vi "test_TxUDPBlockWrite.vi"() -> ()   [LabVIEW 2020]
uses:
  <instrlib>/AIM GmbH/_AIM 664/_controls/port_configuration.ctl
  <instrlib>/AIM GmbH/_AIM 664/_controls/port_speed.ctl
  <instrlib>/AIM GmbH/_AIM 664/_controls/comm_config_vl_tx.ctl
  <instrlib>/AIM GmbH/_AIM 664/_controls/comm_udp_tx.ctl
  <instrlib>/AIM GmbH/_AIM 664/helpers/EthFrameManagement/controls/arinc664_mac_src_info.ctl
  <instrlib>/AIM GmbH/_AIM 664/_controls/comm_computedMAC-IP.ctl
  <instrlib>/AIM GmbH/_AIM 664/bsp/Fdx Create Session (Tx-UDP Port-Oriented).vi
  <instrlib>/AIM GmbH/_AIM 664/bsp/Transmit/FdxCreateTxVL.vi
  <instrlib>/AIM GmbH/_AIM 664/bsp/Fdx Create UDP Port (TX-CommPort).vi
  <instrlib>/AIM GmbH/_AIM 664/bsp/Fdx Start (Tx).vi
  <instrlib>/AIM GmbH/_AIM 664/bsp/Fdx Stop (Tx).vi
  <instrlib>/AIM GmbH/_AIM 664/AIM664LV.lvlib
  BlockMessage/UdpBlockMessage.lvlib
  <instrlib>/AIM GmbH/_AIM 664/bsp/Fdx Create Session (Generic-Board).vi
  <instrlib>/AIM GmbH/_AIM 664/helpers/EthFrameManagement/EthFrameManagement.lvlib
panel:
  out "MsgCountOut":u32
  out "MsgCount 2":u32=2
  out "UdpBlockWriteResultArray":u32[](array[numeric])
  out "Waveform Chart":u32(graph)
  out "CurrentIndex":u32
  out "IndexCycleCount":u32
  out "MsgCount":u32
  out "TxStatus":T1 {"TransmitMode" items=["FDX_TX_GENERIC", "FDX_TX_REPLAY", "FDX_TX_INDIVIDUAL"]; "TxStatus" items=["FDX_STAT_STOP", "FDX_STAT_RUN", "FDX_STAT_ERROR", "FDX_STAT_WAIT_F_TRIG"]}
  in  "stop":bool
  out "Array":T2[](array[typedef]) {"MACsrc" format="%.0x"}
  out "Buf":u8[](array[numeric]) format="%.0x"
  in  "Buf Lenght":i32=512
  in  "VlTx":T3={"domainID"=1, "sideID"=1, "locationID"=1, "interfaceID"=1}
  in  "CommPort Config":T4[](array[typedef])=[{"PortType"=enum."FDX_UDP_SAMPLING", "partitionID"=1, "SubVlId"=1, "UdpSrcPort"=24, "UdpDstPort"=23, "SampleRateMs"=64.0, "UdpNumBufMessages"=1, "UdpMaxMessageSize"=512}, {"PortType"=enum."FDX_UDP_SAMPLING", "partitionID"=2, "SubVlId"=2, "UdpSrcPort"=34, "UdpDstPort"=33, "SampleRateMs"=64.0, "UdpNumBufMessages"=1, "UdpMaxMessageSize"=512}, {"PortType"=enum."FDX_UDP_SAMPLING", "partitionID"=3, "SubVlId"=3, "UdpSrcPort"=44, "UdpDstPort"=43, "SampleRateMs"=64.0, "UdpNumBufMessages"=1, "UdpMaxMessageSize"=512}, {"PortType"=enum."FDX_UDP_SAMPLING", "partitionID"=3, "SubVlId"=4, "UdpSrcPort"=54, "UdpDstPort"=53, "SampleRateMs"=64.0, "UdpNumBufMessages"=1, "UdpMaxMessageSize"=512}]
  in  "VL Config":T5[](array[typedef])=[{"VlId"=60, "NumOfSubVl"=4, "rate ms [Bag]"=64, "domainID"=1, "sideID"=1, "locationID"=1, "interfaceID"=1, "NetSelect"=3, "Skew"=0, "MaxFrameLength"=1518, "FrameBufferSize"=0}] {"NetSelect" items=["FDX_TX_FRAME_DLY_A"=0, "FDX_TX_FRAME_DLY_B"=1, "FDX_TX_FRAME_BOTH "=3, "FDX_TX_FRAME_ONLY_A"=4, "FDX_TX_FRAME_ONLY_B "=5]; "interfaceID" format="%.0b"}
  in  "PortMap":u32=1
  out "PortInitOut":T6 {"PortConfig" items=["FDX_SINGLE", "FDX_REDUNDANT"]}
  in  "port":u32
  in  "PortSpeed":T7[](array[typedef])=[0, 0] items=["FDX_100MBIT"=0, "FDX_10MBIT"=1, "FDX_1000MBIT"=5, "FDX_AUTO_100MBIT"=2, "FDX_AUTO_10MBIT"=3]
  in  "PortConfig":T8[](array[typedef])=[0, 0] items=["FDX_SINGLE", "FDX_REDUNDANT"]
  out "timed out":bool
  out "good link":bool
  out "error out":errorcluster
  in  "board":u32
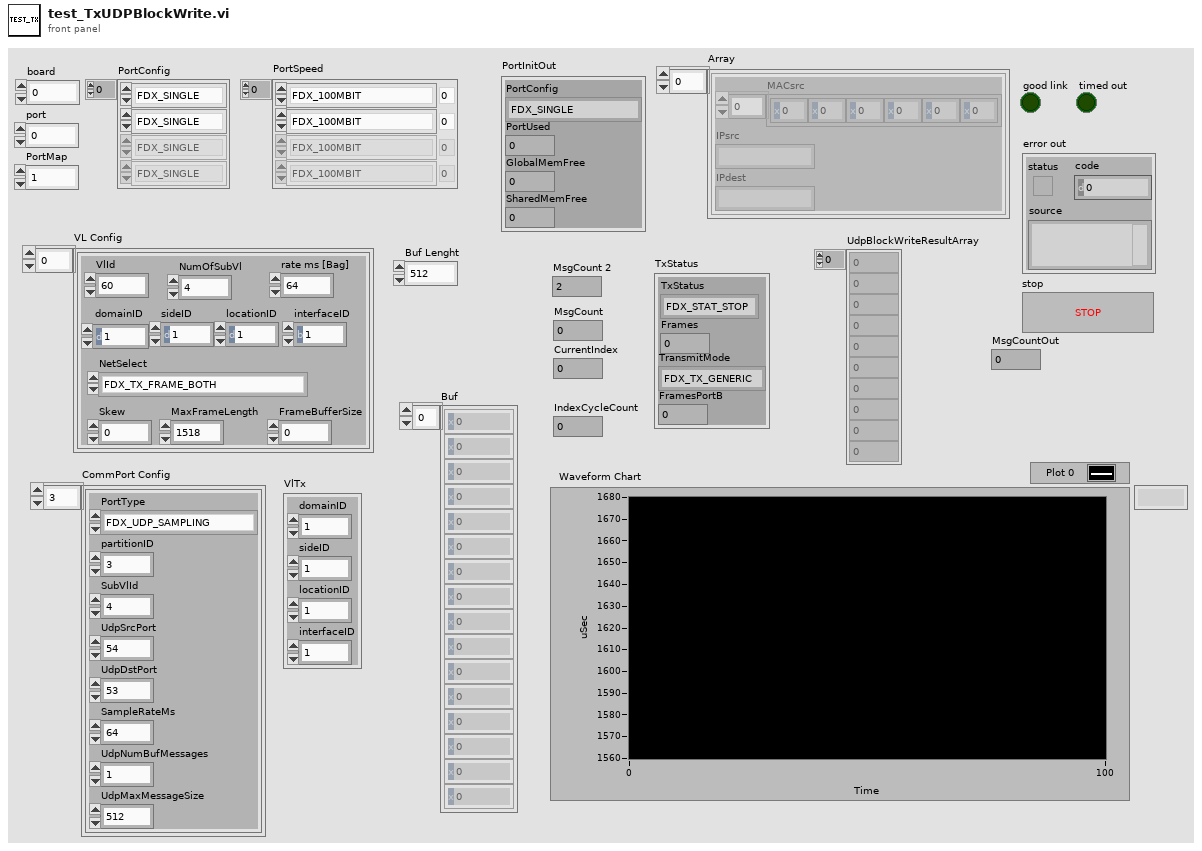
[diagram p1: front panel]
types:
  T1 = cluster{"TxStatus":u32, "Frames":u32, "TransmitMode":u32, "FramesPortB":u32}
  T2 = typedef "AIM664LV.lvlib/comm_computedMAC-IP.ctl" = cluster{"MACsrc":u8[], "IPsrc":string, "IPdest":string}
  T3 = typedef "EthFrameManagement.lvlib/arinc664_mac_src_info.ctl" = cluster{"domainID":u8, "sideID":u8, "locationID":u8, "interfaceID":u8}
  T4 = typedef "AIM664LV.lvlib/comm_udp_tx.ctl" = cluster{"PortType":enum16{"FDX_UDP_SAMPLING", "FDX_UDP_QUEUING"}, "partitionID":u8, "SubVlId":u8, "UdpSrcPort":u16, "UdpDstPort":u16, "SampleRateMs":dbl, "UdpNumBufMessages":u32, "UdpMaxMessageSize":u32}
  T5 = typedef "AIM664LV.lvlib/comm_config_vl_tx.ctl" = cluster{"VlId":u16, "NumOfSubVl":u16, "rate ms [Bag]":u32, "domainID":u8, "sideID":u8, "locationID":u8, "interfaceID":u8, "NetSelect":u32, "Skew":u32, "MaxFrameLength":u32, "FrameBufferSize":u32}
  T6 = cluster{"PortConfig":u32, "PortUsed":u32, "GlobalMemFree":u32, "SharedMemFree":u32}
  T7 = typedef "AIM664LV.lvlib/port_speed.ctl" = u32
  T8 = typedef "AIM664LV.lvlib/port_configuration.ctl" = u32
  T9 = typedef "UdpBlockMessage.lvlib/ubm_value_type.ctl" = cluster{"ul_ByteCount":u32, "ul_UdpHandle":u32, "write index":u32}
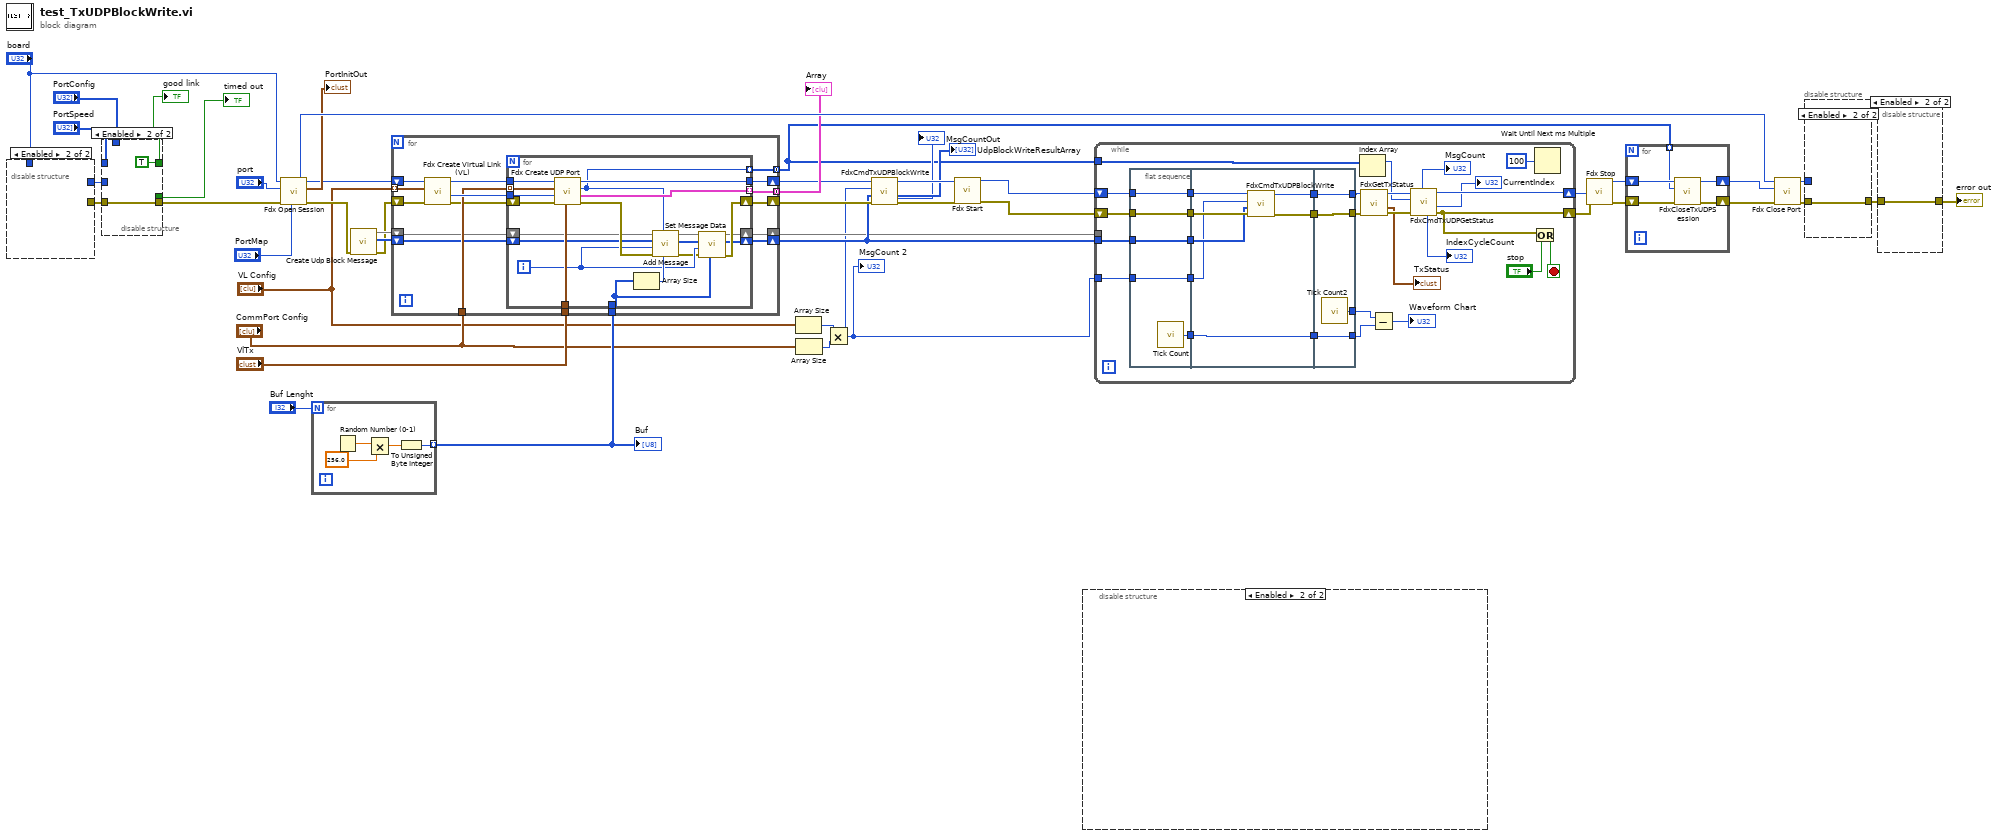
[diagram p0: block diagram]
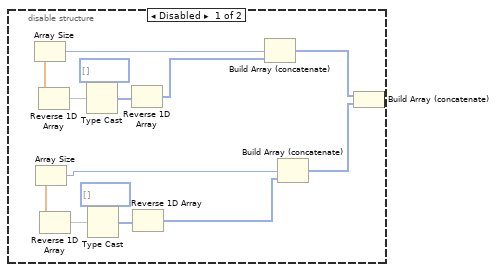
[diagram p2: hidden frame]
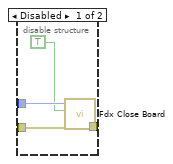
[diagram p3: hidden frame]
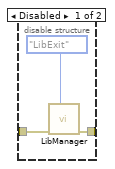
[diagram p4: hidden frame]
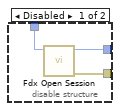
[diagram p5: hidden frame]
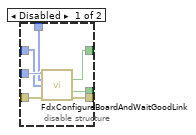
[diagram p6: hidden frame]
diagram:
  n1 = disable-structure shown="Enabled" {
    disable-tunnel: [w50 _] -> w47
    disable-tunnel: [w49 _] -> w46
    disable-tunnel: "board" -> [w48 _]
    frame Disabled {
      n2 = call-poly <instrlib>:"Fdx Open Session.vi"("board"=w48) -> ("error out"=w49:errorcluster, "InstrumentHandle_board out"=w50:u32)  [unwired: 8 in, 1 out]
    }
    frame Enabled {
    }
  }
  n3 = disable-structure shown="Enabled" {
    disable-tunnel: w47 -> [w57 _]
    disable-tunnel: w46 -> [w56 w59]
    disable-tunnel: [w55 TRUE ("good link")] -> w45
    disable-tunnel: [w54 _] -> w44
    disable-tunnel: "PortConfig" -> [w53 _]
    disable-tunnel: "PortSpeed" -> [w52 _]
    disable-tunnel: [w51 w59] -> w41
    frame Disabled {
      n4 = call <instrlib>:"FdxConfigureBoardAndWaitGoodLink.vi"("InstrumentHandle_board in"=w57, "PortConfig"=w53, "PortSpeed"=w52, "error in"=w56) -> ("good link"=w55:bool, "timed out"=w54:bool, "error out"=w51:errorcluster)  [unwired: 8 in, 1 out]
    }
    frame Enabled {
    }
  }
  "good link" <- w45
  "timed out" <- w44
  n5 = call-poly <instrlib>:"Fdx Open Session.vi"("PortMap"="PortMap", "error in (no error)"=w41, "port"="port", "board"="board") -> ("error out"=w7:errorcluster, "PortInitOut"=→"PortInitOut":T6, "port handle out"=w31:u32, "InstrumentHandle_board out"=w36:u32)  [unwired: 3 in, 1 out]
  n6 = for {
    N: "Buf Lenght" -> [_]
    tunnel: [w60] -> w12 mode=indexing
    n7 = Random Number (0-1)() -> (number: 0 to 1=w63:dbl)
    n8 = Multiply(x=w63, y=256.0) -> (x*y=w61:dbl)
    n9 = To Unsigned Byte Integer(number=w61) -> (unsigned 8bit integer=w60:u8)
  }
  "Buf" <- w12
  n10 = call "Create Udp Block Message.vi"("error in (no error)"=w7) -> ("error out"=w4:errorcluster, "Message Block Array"=w5:u32[], "Udp Block Message Map"=w6:map{i32, T9})  [unwired: 8 in]
  n11 = for {
    tunnel: "VL Config" -> [w78] mode=indexing
    tunnel: "VlTx" -> [w75]
    tunnel: [w74] -> w29 mode=concatenating
    tunnel: [w71] -> w13 mode=concatenating
    tunnel: w12 -> [w70]
    tunnel: "CommPort Config" -> [w67]
    shift-right: [w72] -> w18
    shift-left: w4 -> [w80]
    shift-right: [w73] -> w20
    shift-left: w31 -> [w79]
    shift-right: [w68] -> w10
    shift-left: w6 -> [w65]
    shift-right: [w69] -> w11
    shift-left: w5 -> [w64]
    n12 = call-poly <instrlib>:"Fdx Create Virtual Link (VL).vi"("error in (no error)"=w80, "VL Config"=w78, "InstrumentHandle in"=w79) -> ("error out"=w66:errorcluster, "VlId"=w76:u16, "InstrumentHandle out"=w77:u32)  [unwired: 6 in]
    n13 = for {
      tunnel: w77 -> [w100]
      tunnel: w76 -> [w99]
      tunnel: w67 -> [w97] mode=indexing
      tunnel: w75 -> [w96]
      tunnel: [w95] -> w74 mode=indexing
      tunnel: [w94] -> w73
      tunnel: [w90] -> w71 mode=indexing
      shift-right: [w83] -> w72
      shift-left: w66 -> [w98]
      shift-right: [w81] -> w69
      shift-left: w64 -> [w89]
      shift-right: [w82] -> w68
      shift-left: w65 -> [w92]
      tunnel: w70 -> [w88]
      i -> [w87]
      n14 = call-poly <instrlib>:"Fdx Create UDP Port.vi"("VlTx"=w96, "error in"=w98, "VlId"=w99, "CommPort Config"=w97, "port handle in"=w100) -> ("error out"=w93:errorcluster, "computedAddresses"=w95:T2, "commPort handle out"=w90:u32, "port handle out"=w94:u32)  [unwired: 3 in]
      n15 = Array Size(array=w88) -> (size(s)=w91:i32)
      n16 = call "Add Message.vi"("ul_ByteCount"=w91, "ul_UdpHandle"=w90, "error in (no error)"=w93, "index"=w87, "Message Block Array in"=w89, "Udp Block Message Map in"=w92) -> ("error out"=w84:errorcluster, "Message Block Array out"=w85:u32[], "Udp Block Message Map out"=w86:map{i32, T9})  [unwired: 3 in]
      n17 = call "Set Message Data.vi"("Data in"=w88, "error in (no error)"=w84, "index"=w87, "Message Block Array in"=w85, "Udp Block Message Map in"=w86) -> ("error out"=w83:errorcluster, "Message Block Array out"=w81:u32[], "Udp Block Message Map out"=w82:map{i32, T9})  [unwired: 4 in]
    }
  }
  "Array" <- w29
  n18 = Array Size(array="VL Config") -> (size(s)=w1:i32)
  n19 = Array Size(array="CommPort Config") -> (size(s)=w9:i32)
  n20 = Multiply(x=w1, y=w9) -> (x*y=w2:i32)
  "MsgCount 2" <- w2
  n21 = call <instrlib>:"FdxCmdTxUDPBlockWrite.vi"("error in"=w18, "UdpBlockWriteMsgArray"=w11, "MsgCount"=w2, "InstrumentHandle"=w20) -> ("error out"=w17:errorcluster, "UdpBlockWriteResultArray"=→"UdpBlockWriteResultArray":u32[], "InstrumentHandle"=w19:u32, "MsgCountOut"=→"MsgCountOut":u32)  [unwired: 3 in, 1 out]
  n22 = call-poly <instrlib>:"Fdx Start.vi"("error in"=w17, "InstrumentHandle_port in"=w19) -> ("error out"=w28:errorcluster, "InstrumentHandle_port out"=w27:u32)  [unwired: 8 in]
  n23 = disable-structure shown="Enabled" {
    frame Disabled {
      n24 = Array Size() -> (array=w110:dbl[], size(s)=w115:i32)
      n25 = Reverse 1D Array() -> (array=w101:ext[], reversed array=w105:ext[])
      n26 = Array Size(array=w101) -> (size(s)=w102:i32)
      n27 = Reverse 1D Array(array=w110) -> (reversed array=w107:ext[])
      n28 = Type Cast(type=u32[] [] ("Buf"), x=w105) -> (*(type *) &x=w104:u32[])
      n29 = Type Cast(type=u32[] [] ("Buf"), x=w107) -> (*(type *) &x=w108:u32[])
      n30 = Reverse 1D Array(array=w104) -> (reversed array=w106:u32[])
      n31 = Reverse 1D Array(array=w108) -> (reversed array=w116:u32[])
      n32 = Build Array (concatenate)(w102, w106) -> (w111:u32[], w113:u32)
      n33 = Build Array (concatenate)(w115, w116) -> (w112:u32[], w114:u32)
      n34 = Build Array (concatenate)(w111, w112) -> ()  [unwired: 1 out]
    }
    frame Enabled {
    }
  }
  n35 = while {
    shift-right: [w140] -> w25
    shift-left: w27 -> [w134]
    shift-right: [w141] -> w26
    shift-left: w28 -> [w130]
    tunnel: w13 -> [w122]
    tunnel: w11 -> [w119]
    tunnel: w10 -> [_]
    tunnel: w2 -> [w117]
    stop <- w144 stop-if-true
    n36 = flat-sequence {
      tunnel: [w151] -> w135
      tunnel: w134 -> [w151]
      tunnel: [w150] -> w131
      tunnel: w130 -> [w150]
      tunnel: [w149] -> w128
      tunnel: [w148] -> w120
      tunnel: w119 -> [w148]
      tunnel: [w147] -> w118
      tunnel: w117 -> [w147]
      tunnel: w135 -> [w157]
      tunnel: [w154] -> w132
      tunnel: w131 -> [w156]
      tunnel: [w158] -> w129
      tunnel: w128 -> [w158]
      tunnel: [w155] -> w123
      tunnel: w120 -> [w153]
      tunnel: w118 -> [w152]
      tunnel: [w162] -> w133
      tunnel: w132 -> [w162]
      tunnel: [w161] -> w127
      tunnel: [w160] -> w126
      tunnel: w129 -> [w160]
      tunnel: [w159] -> w124
      tunnel: w123 -> [w159]
      frame #0 {
        n37 = call "Tick Count"() -> ("Tick Count(uSec)"=w149:u32)
      }
      frame #1 {
        n38 = call <instrlib>:"FdxCmdTxUDPBlockWrite.vi"("error in"=w156, "UdpBlockWriteMsgArray"=w153, "MsgCount"=w152, "InstrumentHandle"=w157) -> ("error out"=w155:errorcluster, "InstrumentHandle"=w154:u32)  [unwired: 3 in, 3 out]
      }
      frame #2 {
        n39 = call "Tick Count2"() -> ("Tick Count(uSec)"=w161:u32)
      }
    }
    n40 = Index Array(array=w122) -> (element=w121:u32)  [unwired: 1 in]
    n41 = call <instrlib>:"FdxGetTxStatus.vi"("error in"=w124, "InstrumentHandle_port"=w133) -> ("error out"=w143:errorcluster, "TxStatus"=→"TxStatus":T1, "InstrumentHandle_port"=w142:u32)  [unwired: 7 in]
    n42 = Subtract(x=w127, y=w126) -> (x-y=→"Waveform Chart":u32)
    n43 = call <instrlib>:"FdxCmdTxUDPGetStatus.vi"("error in"=w143, "UdpHandle"=w121, "InstrumentHandle"=w142) -> ("error out"=w141:errorcluster, "CurrentIndex"=→"CurrentIndex":u32, "InstrumentHandle"=w140:u32, "IndexCycleCount"=→"IndexCycleCount":u32, "MsgCount"=→"MsgCount":u32)  [unwired: 3 in, 1 out]
    n44 = Or(x=w141, y="stop") -> (x .or. y?=w144:bool)
    n45 = Wait Until Next ms Multiple(millisecond multiple=u32 100) -> ()  [unwired: 1 out]
  }
  n46 = call-poly <instrlib>:"Fdx Stop.vi"("error in"=w26, "InstrumentHandle_port in"=w25) -> ("error out"=w24:errorcluster, "InstrumentHandle_port out"=w21:u32)  [unwired: 8 in]
  n47 = for {
    tunnel: w13 -> [w163] mode=indexing
    shift-right: [w166] -> w23
    shift-left: w24 -> [w167]
    shift-right: [w165] -> w22
    shift-left: w21 -> [w164]
    n48 = call <instrlib>:"FdxCloseTxUDPSession.vi"("error in"=w167, "UdpHandle"=w163, "InstrumentHandle"=w164) -> ("error out"=w166:errorcluster, "InstrumentHandle"=w165:u32)  [unwired: 7 in]
  }
  n49 = call <instrlib>:"Fdx Close Port.vi"("error in"=w23, "InstrumentHandle_port in"=w22, "InstrumentHandle_board in"=w36) -> ("error out"=w38:errorcluster, "InstrumentHandle_board out"=w37:u32)  [unwired: 7 in]
  n50 = disable-structure shown="Enabled" {
    disable-tunnel: w38 -> [w171 w172]
    disable-tunnel: w37 -> [w170 _]
    disable-tunnel: [w168 w172] -> w33
    frame Disabled {
      n51 = call <instrlib>:"Fdx Close Board.vi"("error in"=w171, "Force Board Release (F)"=TRUE ("Close reference to library?"), "InstrumentHandle_board in"=w170) -> ("error out"=w168:errorcluster)  [unwired: 8 in]
    }
    frame Enabled {
    }
  }
  n52 = disable-structure shown="Enabled" {
    disable-tunnel: w33 -> [w174 w176]
    disable-tunnel: [w173 w176] -> w32
    frame Disabled {
      n53 = call <instrlib>:"LibManager.vi"("action"=enum16{"LibInit", "LibExit"}."LibExit", "error in (no error)"=w174) -> ("error out"=w173:errorcluster)  [unwired: 7 in, 2 out]
    }
    frame Enabled {
    }
  }
  "error out" <- w32
